vi "HowdyDrive.vi"(6 "highGear?":bool, 8 "error in (no error)":errorcluster, 9 "Y":dbl, 10 "X":dbl, 11 "Drive in":refnum<class "Drive.lvclass">) -> (0 "error out":errorcluster, 3 "Drive out":refnum<class "Drive.lvclass">)   [LabVIEW 2019, in "DriveOld.lvlib" / "Drive.lvclass"]
doc: "Runs motors based of joystick values in velocity closed loop mode, a version of arcade drive with support for CTRE motor controllers"
uses:
  Drive.lvclass
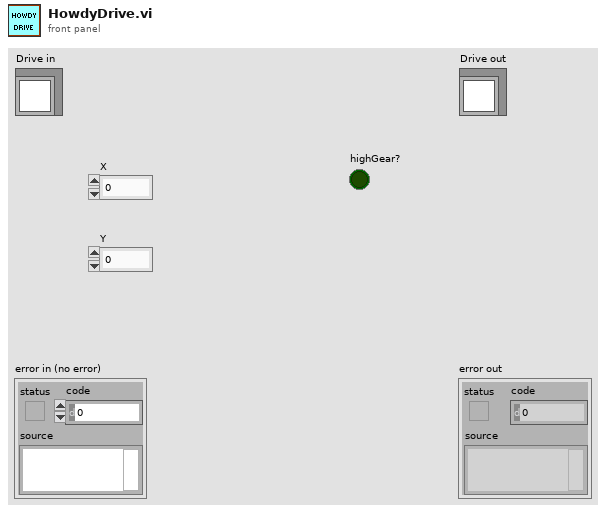
[diagram p1: front panel]
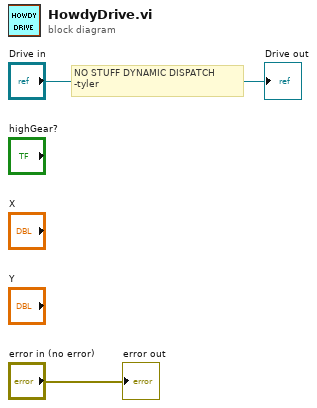
[diagram p0: block diagram]
diagram:
  # "NO STUFF DYNAMIC DISPATCH\n-tyler"
  "error out" <- "error in (no error)"
  "Drive out" <- "Drive in"
